vi "Digital Read.vi"   [LabVIEW 2011, in "LMH-LINX.lvlib"]
doc: "Read the value of the specified digital input channel(s)."
uses:
  LMH-LINX.lvlib
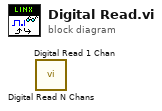
[diagram p0: block diagram]
diagram:
  n1 = call "Digital Read N Chans.vi"() -> ()  [unwired: 9 in, 3 out]
  n2 = call "Digital Read 1 Chan.vi"() -> ()  [unwired: 9 in, 3 out]
